vi "HandShaking.vi"(6 "Elapsed Time":u32, 8 "error in (no error)":errorcluster, 10 "Event Sources":T1, 11 "PreUUT in":refnum<class "PreUUT.lvclass">) -> (0 "error out":errorcluster, 3 "PreUUT out":refnum<class "PreUUT.lvclass">)   [LabVIEW 2021, in "PreUUT.lvclass"]
uses:
  PreUUT.lvclass
  PreUUT.lvclass/PreUUT.ctl
  OPC UA/OPC UA.lvclass
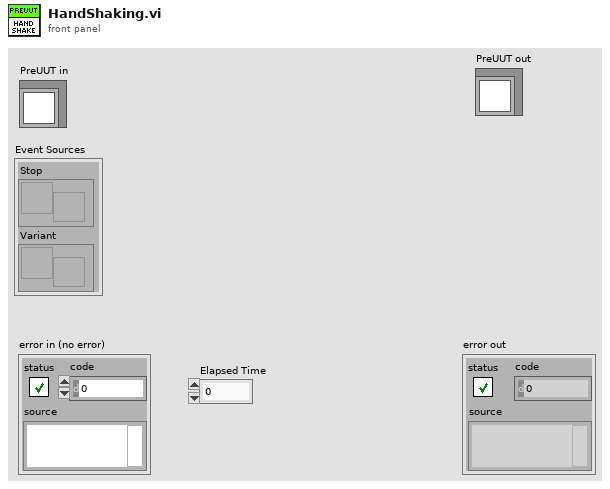
[diagram p1: front panel]
types:
  T1 = cluster{"Stop":refnum<user-event>, "Variant":refnum<user-event>}
  T2 = typedef "PreUUT.lvclass/Rx PreUUT.ctl" = cluster{"NestStatus":bool, "PalletID":u32, "Start":bool, "BarcodeData":string, "FaultCode":u32, "Stop":bool}
  T3 = typedef "PreUUT.lvclass/Tx PreUUT.ctl" = cluster{"Online":bool, "Ready":bool, "Fault":bool, "Timeout":bool, "Results":u32, "StepNo":u32, "TestRunning":bool, "ResultsReady":bool}
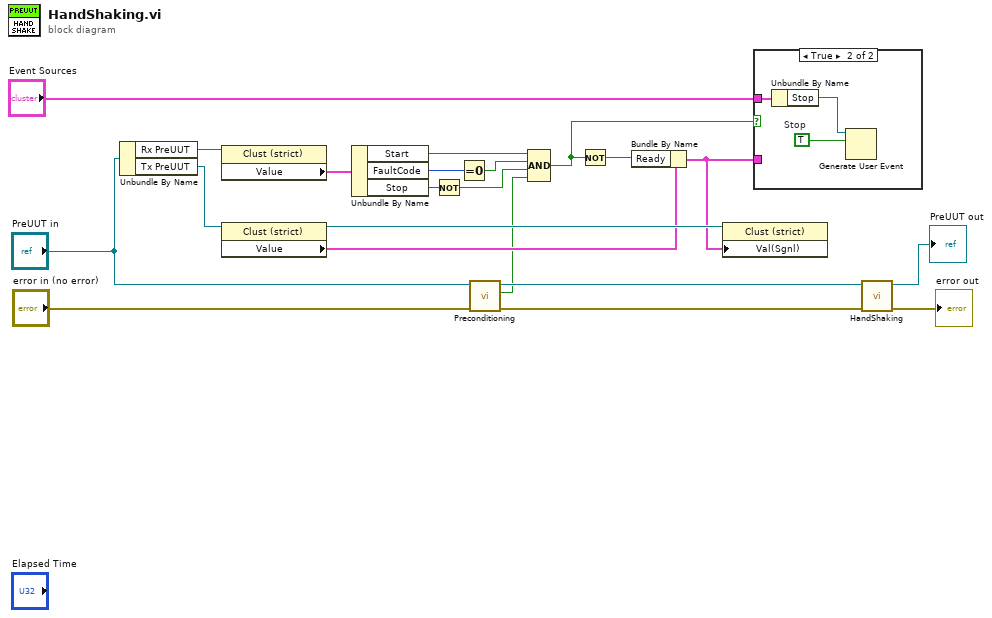
[diagram p0: block diagram]
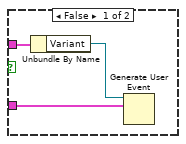
[diagram p2: hidden frame]
diagram:
  n1 = Unbundle By Name("PreUUT in") -> ("Rx PreUUT"=w19:refnum<vi>, "Tx PreUUT"=w9:refnum<vi>)
  n2 = property class="Clust (strict)"(reference=w19) -> ("Value"=w10:T2)  [unwired: 1 in, 2 out]
  n3 = property class="Clust (strict)"(reference=w9) -> (reference out=w20:refnum<vi>, "Value"=w18:T3)  [unwired: 1 in, 1 out]
  n4 = Unbundle By Name(w10) -> ("Start"=w11:bool, "FaultCode"=w13:u32, "Stop"=w14:bool)
  n5 = Not(x=w14) -> (.not. x?=w15:bool)
  n6 = Equal To 0?(x=w13) -> (x = 0?=w12:bool)
  n7 = call "Preconditioning.vi"("error in (no error)"="error in (no error)", "PreUUT in"="PreUUT in") -> ("error out"=w1:errorcluster, "Preconditioning"=w4:bool, "PreUUT out"=w5:refnum<class "PreUUT.lvclass">)  [unwired: 7 in]
  n8 = Compound Arithmetic op=AND(w11, w12, w15, w4) -> (w2:bool)
  n9 = Not(x=w2) -> (.not. x?=w17:bool)
  n10 = Bundle By Name(cluster=w18, "Ready"=w17) -> (w3:T3)
  n11 = property class="Clust (strict)"(reference=w20, "Val(Sgnl)"=w3) -> ()  [unwired: 1 in, 2 out]
  n12 = case shown="True" w2 {
    tunnel: w3 -> [w24 _]
    tunnel: "Event Sources" -> [w23 w27]
    frame False {
      n13 = Unbundle By Name(w23) -> ("Variant"=w22:refnum<user-event>)
      n14 = Generate User Event(user event=w22, event data cluster=w24) -> ()  [unwired: 2 in, 2 out]
    }
    frame True {
      w25 = TRUE  # Stop
      n15 = Unbundle By Name(w27) -> ("Stop"=w26:refnum<user-event>)
      n16 = Generate User Event(user event=w26, event data cluster=w25) -> ()  [unwired: 2 in, 2 out]
    }
  }
  n17 = call-parent "HandShaking.vi"("error in (no error)"=w1, "OPC UA in"=w5) -> ("error out"=→"error out":errorcluster, "OPC UA out"=→"PreUUT out":refnum<class "PreUUT.lvclass">)  [unwired: 8 in]
